vi "example_dispersion.vi"() -> ()   [LabVIEW 2015]
panel:
  in  "disp":enum32{"Absorption", "Dispersion"}(ring)=enum."Dispersion" caption="disp (Absorption)"
  in  "nu":dbl=112266.5949 format="%#_13g"
  in  "alpha":dbl=1.98573285442 caption="alpha (10)" format="%#_13g"
  in  "Ylm":dbl=0.0005 caption="Ylm (0)" format="%#_13g"
  in  "Xlm":dbl=0.001 caption="Xlm (0)" format="%#_13g"
  in  "GammaD":dbl=0.0351 caption="GammaD (0)" format="%#_13g"
  in  "nu0":dbl=112265.5949 caption="nu0 (0)" format="%#_13g"
  in  "NuOptIm":dbl=-0.0175 caption="NuOptIm (0)" format="%#_13g"
  in  "NuOptRe":dbl=0.038 caption="NuOptRe (0)" format="%#_13g"
  in  "Delta2":dbl=0.0124 caption="Delta2 (0)" format="%#_13g"
  in  "Gamma2":dbl=0.0054 caption="Gamma2 (0)" format="%#_13g"
  in  "Delta0":dbl=0.0305 caption="Delta0 (0)" format="%#_13g"
  in  "Gamma0":dbl=0.0117 caption="Gamma0 (0)" format="%#_13g"
  out "mHT":dbl=-0.32897836537038816 format="%#_16g"
  # "Input Section"
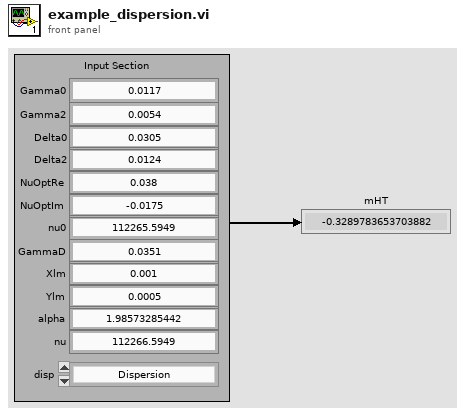
[diagram p1: front panel]
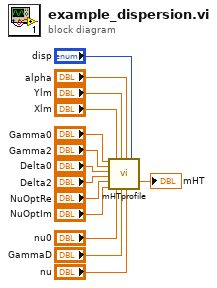
[diagram p0: block diagram]
diagram:
  n1 = call "mHTprofile.vi"("Gamma0"="Gamma0", "Gamma2"="Gamma2", "Delta0"="Delta0", "Delta2"="Delta2", "NuOptRe"="NuOptRe", "NuOptIm"="NuOptIm", "Xlm"="Xlm", "nu0"="nu0", "Ylm"="Ylm", "GammaD"="GammaD", "alpha"="alpha", "nu"="nu", "disp"="disp") -> ("mHT"=→"mHT":dbl)  [unwired: 6 in]
